vi "medidorIXV.vi"() -> (0 "tempo de medicao":dbl, 2 "Corrente Atual":dbl, 3 "Tensao Atual":dbl)   [LabVIEW 2012]
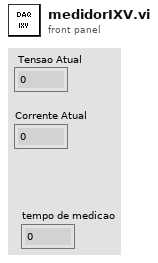
[diagram p1: front panel]
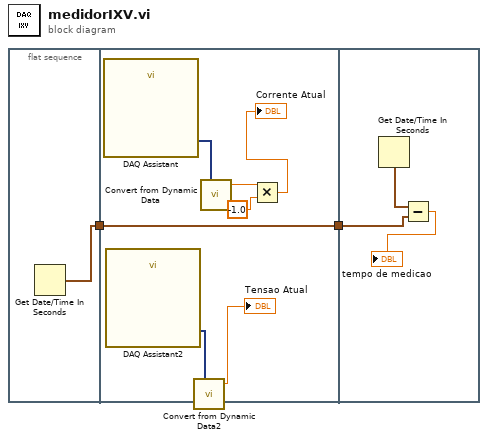
[diagram p0: block diagram]
diagram:
  n1 = flat-sequence {
    tunnel: [w3] -> w1
    tunnel: [w4] -> w2
    tunnel: w1 -> [w4]
    tunnel: w2 -> [w11]
    frame #0 {
      n2 = Get Date/Time In Seconds() -> (seconds since 1Jan1904=w3:timestamp)
    }
    frame #1 {
      n3 = call "DAQ Assistant"() -> ("data"=w8:dynamicdata)  [unwired: 17 in, 2 out]
      n4 = call "DAQ Assistant2"() -> ("data"=w10:dynamicdata)  [unwired: 17 in, 2 out]
      n5 = call "Convert from Dynamic Data2"("Dynamic Data Type"=w10) -> ("Scalar"=→"Tensao Atual":dbl)  [unwired: 3 in]
      n6 = call "Convert from Dynamic Data"("Dynamic Data Type"=w8) -> ("Scalar"=w6:dbl)  [unwired: 3 in]
      n7 = Multiply(x=w6, y=-1.0) -> (x*y=→"Corrente Atual":dbl)
    }
    frame #2 {
      n8 = Get Date/Time In Seconds() -> (seconds since 1Jan1904=w12:timestamp)
      n9 = Subtract(x=w12, y=w11) -> (x-y=→"tempo de medicao":dbl)
    }
  }
